vi "Get EDS.vi"(10 "Path":path, 11 "UI Actor in":refnum<class "UI Actor.lvclass">) -> (2 "EDS":refnum<class "EDS.lvclass">, 3 "UI Actor out":refnum<class "UI Actor.lvclass">)   [LabVIEW 2024, in "UI Actor.lvlib" / "UI Actor.lvclass"]
uses:
  UI Actor.lvclass
  UI Actor.lvclass/UI Actor.ctl
  Core/EDS/EDS.lvclass
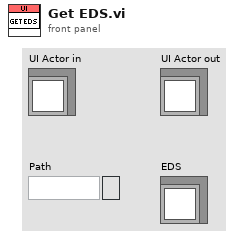
[diagram p1: front panel]
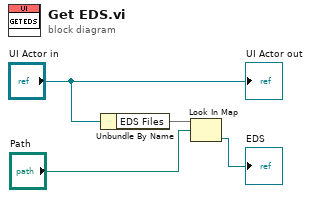
[diagram p0: block diagram]
diagram:
  n1 = Unbundle By Name("UI Actor in") -> ("EDS Files"=w3:map{path, refnum<class "EDS.lvclass">})
  n2 = Look In Map(map=w3, key="Path") -> (value=→"EDS":refnum<class "EDS.lvclass">)  [unwired: 1 in, 1 out]
  "UI Actor out" <- "UI Actor in"
